vi "Get Block Size.vi"(11 "Hash Function in":refnum<class "NI_SHA-512.lvclass">) -> (2 "block size (bytes)":i32, 3 "Hash Function out":refnum<class "NI_SHA-512.lvclass">)   [LabVIEW 2020, in "NI_SHA-512.lvclass"]
uses:
  <vilib>/security/Message Digest/SHA-2/SHA-512/NI_SHA-512.lvclass
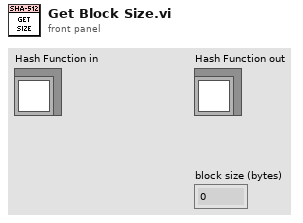
[diagram p1: front panel]
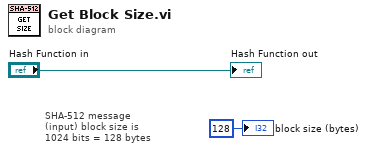
[diagram p0: block diagram]
diagram:
  # "SHA-512 message (input) block size is 1024 bits = 128 bytes"
  "Hash Function out" <- "Hash Function in"
  "block size (bytes)" <- 128 ("block size (bytes)")
